vi "Write CAN Port Configuration.vi"(8 "error in (no error)":errorcluster, 10 "CAN Port Configuration":refnum<data-value>, 11 "Performanced XNET CAN Signal Logger in":refnum<class "Performanced XNET CAN Signal Logger.lvclass">) -> (0 "error out":errorcluster, 3 "Performanced XNET CAN Signal Logger out":refnum<class "Performanced XNET CAN Signal Logger.lvclass">)   [LabVIEW 2021, in "Performanced XNET CAN Signal Logger.lvlib" / "Performanced XNET CAN Signal Logger.lvclass"]
uses:
  Performanced XNET CAN Signal Logger.lvclass
  Typedef/Def-CAN Port Configuration.ctl
  Performanced XNET CAN Signal Logger.lvclass/Performanced XNET CAN Signal Logger.ctl
  XNET-CAN-Signal-Logger.lvlib
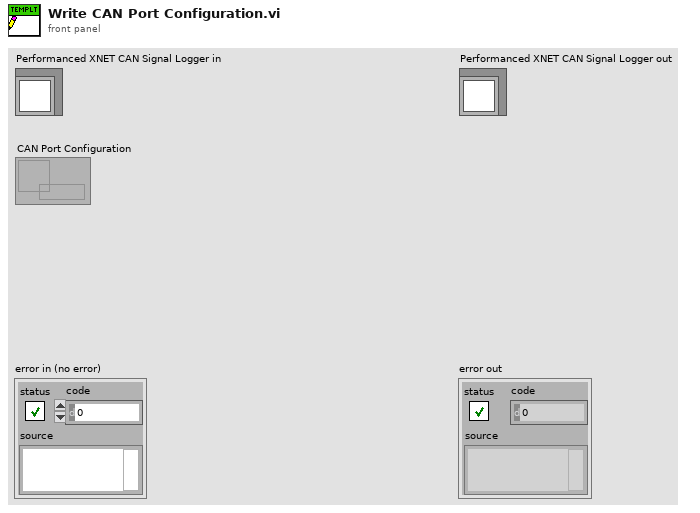
[diagram p1: front panel]
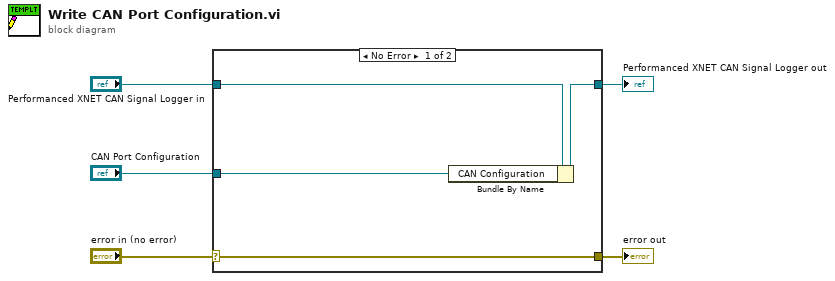
[diagram p0: block diagram]
diagram:
  n1 = case shown="No Error" "error in (no error)" {
    selector: "error in (no error)" -> [w9 w10]
    tunnel: [w9 w10] -> w4
    tunnel: [w7 w11] -> w2
    tunnel: "Performanced XNET CAN Signal Logger in" -> [w8 w11]
    tunnel: "CAN Port Configuration" -> [w6 _]
    frame No Error {
      n2 = Bundle By Name(cluster=w8, "CAN Configuration"=w6) -> (w7:refnum<class "Performanced XNET CAN Signal Logger.lvclass">)
    }
    frame Error {
    }
  }
  "error out" <- w4
  "Performanced XNET CAN Signal Logger out" <- w2
